vi "Save_Config.vi"(8 "Error In":errorcluster, 11 "Data":T1={"Info Box"="", "MAC & Name Out"=[], "Default Gateway"="", "Drfiter IP Addresses"=[], "Network Map"="", "Drifter Selection"=0, "File Selection"=0, "Download File Path"=path "", "File Selection Strings"=[], "Sample Rate"=enum." 0.2", "Log While Charging"=enum." Yes"}) -> (0 "Error Out":errorcluster, 3 "File Contents":string)   [LabVIEW 2017]
uses:
  data.ctl
  <vilib>/httpClient/LabVIEWHTTPClient.lvlib
panel:
  out "body":string
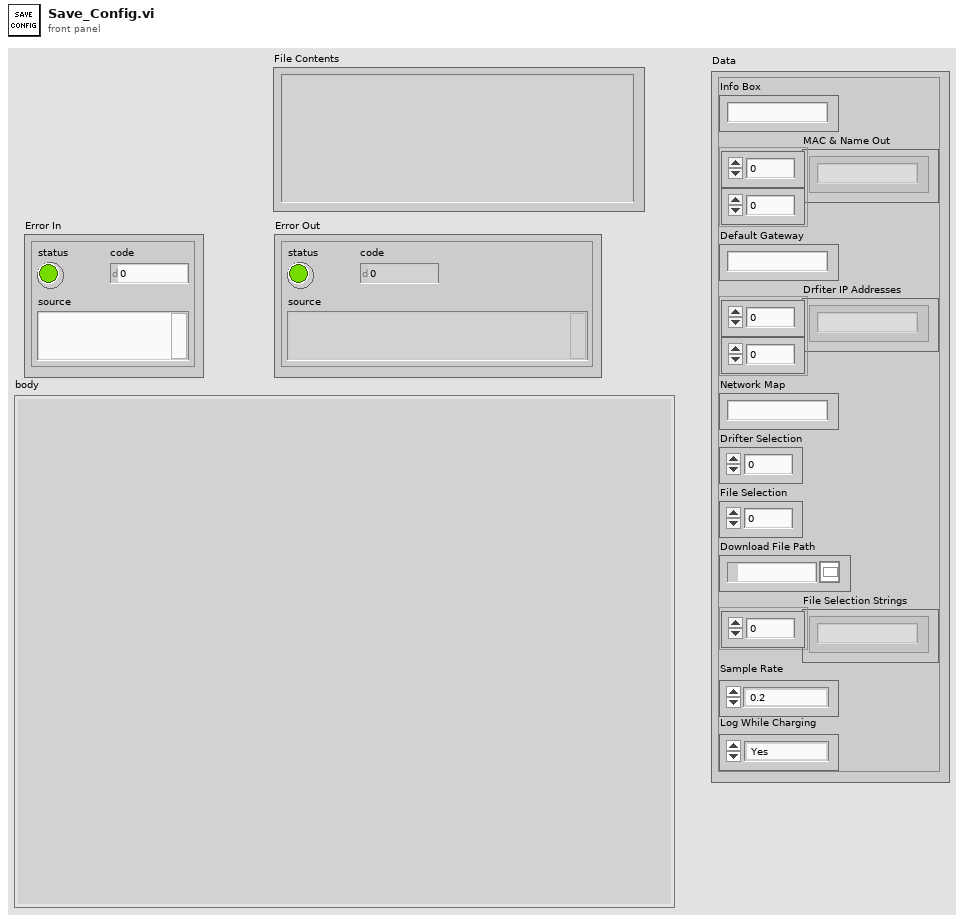
[diagram p1: front panel]
types:
  T1 = typedef "data.ctl" = cluster{"Info Box":string, "MAC & Name Out":string[][], "Default Gateway":string, "Drfiter IP Addresses":string[][], "Network Map":string, "Drifter Selection":i32, "File Selection":i32, "Download File Path":path, "File Selection Strings":string[], "Sample Rate":enum32{"No Selection", " 0.2", " 0.1", " 1", " 2", " 5", " 10"}, "Log While Charging":enum32{"No Selection", " Yes", " No"}}
  T2 = cluster{"Name":string, "Value":string, "appended path":path, "Filename":string, "MIME type":string}
  T3 = cluster{"Name":string, "Value":string, "appended path":path, "Filename":string, "MIME type":string}[]
  T4 = typedef "LabVIEWHTTPClient.lvlib/ClientHandle.ctl" = refnum<k1>
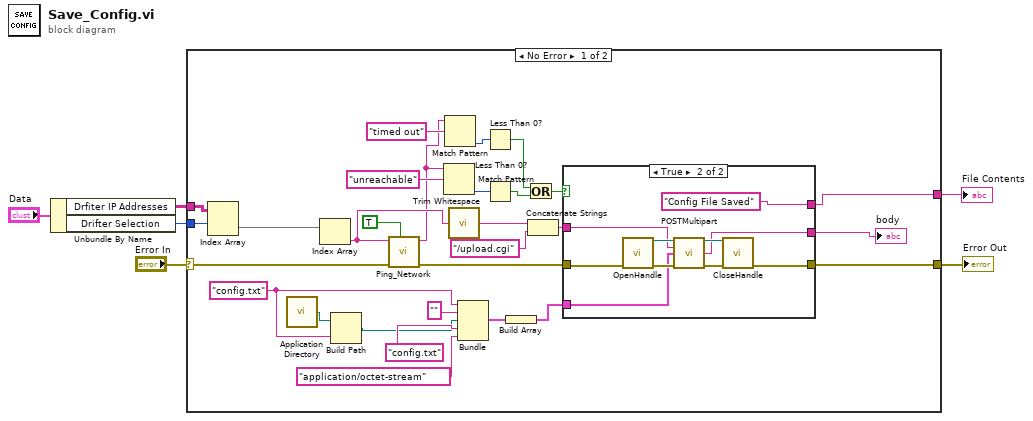
[diagram p0: block diagram]
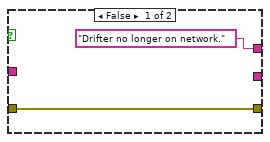
[diagram p2: hidden frame]
diagram:
  n1 = Unbundle By Name("Data") -> ("Drfiter IP Addresses"=w4:string[][], "Drifter Selection"=w3:i32)
  n2 = case shown="No Error" "Error In" {
    selector: "Error In" -> [w27 w48]
    tunnel: [w35 w48] -> w5
    tunnel: w4 -> [w29 _]
    tunnel: w3 -> [w26 _]
    tunnel: [w23 _] -> w1
    frame No Error {
      w14 = "config.txt" ("Name")
      n3 = Index Array(array=w29, index (row)=w26) -> (element=w34:string[])  [unwired: 1 in]
      n4 = call <vilib>:"Application Directory.vi"() -> ("Application Directory"=w13:path)
      n5 = Index Array(array=w34) -> (element=w28:string)  [unwired: 1 in]
      n6 = Build Path(base path=w13, name or relative path=w14) -> (appended path=w15:path)
      n7 = call "Ping_Network.vi"("IP/Default Gateway (T/F)"=TRUE, "Error In"=w27, "Default Gateway/IP"=w28) -> ("Error Out"=w30:errorcluster, "Terminal Output"=w9:string)  [unwired: 7 in]
      n8 = Match Pattern(string=w9, regular expression="unreachable") -> (offset past match=w31:i32)  [unwired: 1 in, 3 out]
      n9 = Match Pattern(string=w9, regular expression="timed out") -> (offset past match=w11:i32)  [unwired: 1 in, 3 out]
      n10 = call <vilib>:"Trim Whitespace.vi"("string"=w28) -> ("trimmed string"=w25:string)  [unwired: 1 in]
      n11 = Bundle("Name"=w14, "Value"="", "appended path"=w15, "Filename"="config.txt", "MIME type"="application/octet-stream") -> (w19:T2)  [unwired: 1 in]
      n12 = Less Than 0?(x=w11) -> (x < 0?=w12:bool)
      n13 = Less Than 0?(x=w31) -> (x < 0?=w7:bool)
      n14 = Build Array(w19) -> (w17:T3)
      n15 = Or(x=w12, y=w7) -> (x .or. y?=w8:bool)
      n16 = Concatenate Strings(w25, "/upload.cgi" ("string")) -> (w18:string)
      n17 = case shown="True" w8 {
        tunnel: w30 -> [w37 w41]
        tunnel: [w37 w42] -> w35
        tunnel: ["Drifter no longer on network." ("Body") "Config File Saved" ("Body")] -> w23
        tunnel: w18 -> [_ w40]
        tunnel: w17 -> [_ w39]
        tunnel: [_ w38] -> w16
        frame False {
        }
        frame True {
          n18 = call <vilib>:"OpenHandle.vi"("error in (no error)"=w41) -> ("client handle out"=w43:T4, "error out"=w44:errorcluster)  [unwired: 13 in]
          n19 = call <vilib>:"POSTMultipart.vi"("client handle"=w43, "url"=w40, "data"=w39, "error in (no error)"=w44) -> ("client handle out"=w45:T4, "body"=w38:string, "error out"=w46:errorcluster)  [unwired: 8 in, 1 out]
          n20 = call <vilib>:"CloseHandle.vi"("client handle"=w45, "error in (no error)"=w46) -> ("error out"=w42:errorcluster)  [unwired: 13 in]
        }
      }
      "body" <- w16
    }
    frame Error {
    }
  }
  "Error Out" <- w5
  "File Contents" <- w1
